vi "Configure LocalQueue Server.vi"(6 "timeout (500 ms)":i32=500, 8 "error in (no error)":errorcluster, 11 "Queue Name":string) -> (0 "error out":errorcluster, 3 "Connection.LocalQueue":refnum<class "Connection.LocalQueue.lvclass">)   [LabVIEW 2013, in "Connection.Queue_GOSPL.lvlib" / "Connection.LocalQueue.lvclass"]
uses:
  Connection.LocalQueue.lvclass
  Connection/Connection.lvclass/Connection.ctl
  Connection/Connection.lvclass
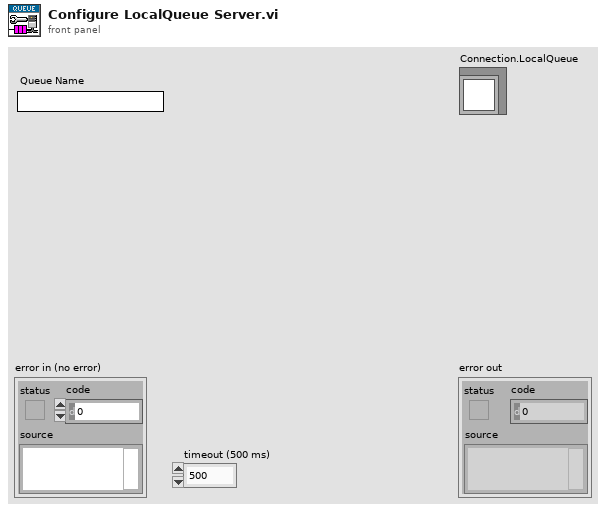
[diagram p1: front panel]
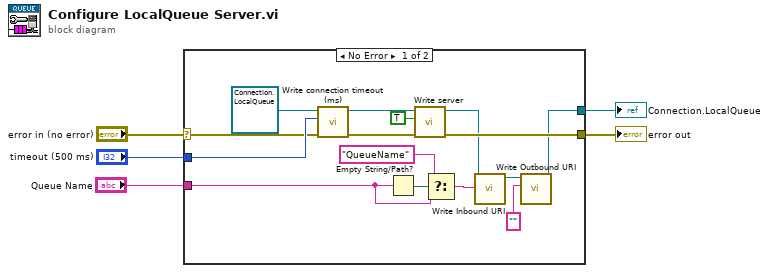
[diagram p0: block diagram]
diagram:
  n1 = case shown="No Error" "error in (no error)" {
    selector: "error in (no error)" -> [w18 w20]
    tunnel: [w17 w20] -> w4
    tunnel: [w7 _] -> w2
    tunnel: "timeout (500 ms)" -> [w19 _]
    tunnel: "Queue Name" -> [w6 _]
    frame No Error {
      n2 = call "Write connection timeout (ms).vi"("error in (no error)"=w18, "connection timeout (ms)"=w19, "Connection in"=refnum<class "Connection.LocalQueue.lvclass"> refnum ("Connection.LocalQueue")) -> ("error out"=w17:errorcluster, "Connection out"=w15:refnum<class "Connection.LocalQueue.lvclass">)  [unwired: 7 in]
      n3 = Empty String/Path?(string/path=w6) -> (empty?=w9:bool)
      n4 = call "Write server.vi"("server"=TRUE, "Connection in"=w15) -> ("Connection out"=w8:refnum<class "Connection.LocalQueue.lvclass">)  [unwired: 9 in]
      n5 = Select(t="QueueName", s=w9, f=w6) -> (s? t:f=w13:string)
      n6 = call "Write Inbound URI.vi"("Inbound URI"=w13, "Connection in"=w8) -> ("Connection out"=w11:refnum<class "Connection.LocalQueue.lvclass">)  [unwired: 9 in]
      n7 = call "Write Outbound URI.vi"("Outbound URI"="" ("Outbound Stream URI"), "Connection in"=w11) -> ("Connection out"=w7:refnum<class "Connection.LocalQueue.lvclass">)  [unwired: 9 in]
    }
    frame Error {
    }
  }
  "error out" <- w4
  "Connection.LocalQueue" <- w2
